vi "mqtt_publisher.vi"() -> ()   [LabVIEW 2024]
uses:
  <vilib>/LabVIEW Open Source Project/Connection/Connection.TCP/Connection.TCP.lvclass
  C:/Program Files (x86)/National Instruments/LabVIEW 2024/vi.lib/LabVIEW Open Source Project/Connection/Connection/Connection.lvclass
  <vilib>/LabVIEW Open Source Project/MQTT Client/Client class/Client.lvclass
  C:/Program Files (x86)/National Instruments/LabVIEW 2024/vi.lib/LabVIEW Open Source Project/MQTT Connection/MQTT_Base/Base Class/MQTT_Base.lvclass
  <vilib>/LabVIEW Open Source Project/MQTT Connection/MQTT_Base/Base Class/MQTT_Base.lvclass
panel:
  out "connected":bool
  in  "stop":bool
  out "Waveform Chart":i32(graph)
  out "last error":errorcluster
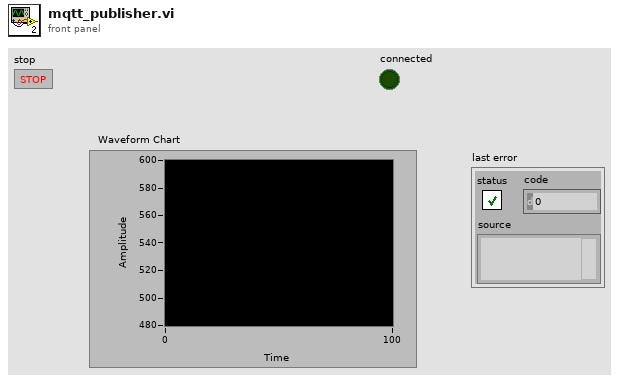
[diagram p1: front panel]
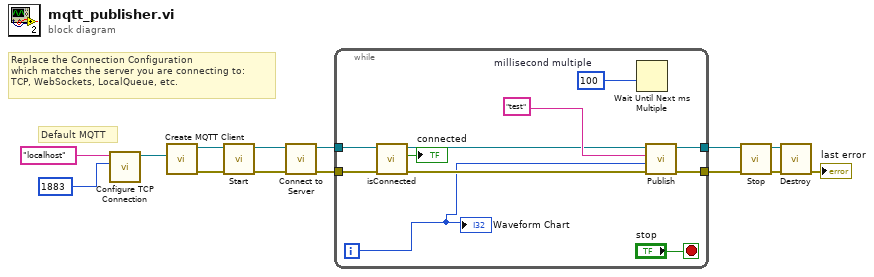
[diagram p0: block diagram]
diagram:
  # "Default MQTT"
  # "Replace the Connection Configuration\nwhich matches the server you are connecting to:\nTCP, WebSockets, LocalQueue, etc."
  n1 = call <vilib>:"Configure TCP Connection.vi"("remote port (80)"=u16 1883, "address (localhost)"="localhost") -> ("Connection.TCP"=w14:refnum<class "Connection.TCP.lvclass">)  [unwired: 8 in, 1 out]
  n2 = call <vilib>:"Create MQTT Client.vi"("Connection Configuration"=w14) -> ("error out"=w7:errorcluster, "Client out"=w8:refnum<class "Client.lvclass">)  [unwired: 9 in]
  n3 = call <vilib>:"Start.vi"("error in (no error)"=w7, "MQTT_Base in"=w8) -> ("error out"=w5:errorcluster, "MQTT_Base out"=w6:refnum<class "Client.lvclass">)  [unwired: 7 in, 1 out]
  n4 = call <vilib>:"Connect to Server.vi"("error in (no error)"=w5, "Client in"=w6) -> ("error out"=w3:errorcluster, "Client out"=w4:refnum<class "Client.lvclass">)  [unwired: 6 in, 2 out]
  n5 = while {
    tunnel: w4 -> [w25]
    tunnel: w3 -> [w24]
    tunnel: [w20] -> w2
    tunnel: [w19] -> w1
    i -> [w15]
    stop <- "stop" stop-if-true
    w17 = u32 100  # millisecond multiple
    n6 = call <vilib>:"isConnected.vi"("error in (no error)"=w24, "Client in"=w25) -> ("error out"=w21:errorcluster, "connected"=→"connected":bool, "Client out"=w22:refnum<class "Client.lvclass">)  [unwired: 7 in]
    n7 = Wait Until Next ms Multiple(millisecond multiple=w17) -> ()  [unwired: 1 out]
    n8 = call <vilib>:"Publish.vi"("error in (no error)"=w21, "Payload"=w15, "Topic Name (empty: Payload name)"="test", "Client in"=w22) -> ("error out"=w19:errorcluster, "Client out"=w20:refnum<class "Client.lvclass">)  [unwired: 5 in, 1 out]
    "Waveform Chart" <- w15
  }
  n9 = call <vilib>:"Stop.vi"("error in (no error)"=w1, "MQTT_Base in"=w2) -> ("error out"=w12:errorcluster, "MQTT_Base out"=w11:refnum<class "Client.lvclass">)  [unwired: 7 in, 1 out]
  n10 = call <vilib>:"Destroy.vi"("error in (no error)"=w12, "MQTT_Base in"=w11) -> ("error out"=→"last error":errorcluster)  [unwired: 8 in, 1 out]
